vi "LVAPT_Git_Item_OnUpdateCommand.vi"(10 "Menu Item In":T1={"Menu Name"="", "Description"="", "Icon File Name"=path "", "Menu Tag"="", "Enabled"=TRUE, "Checked"=FALSE, "Separator"=FALSE, "Batchable"=TRUE, "Weight"=0, "Batch Mode (Ignored if Not Batchable)"=enum."Show If All Items Support Command", "Menu Location"=enum."<None>", "Exclude From Getting Started Window Menu"=FALSE}, 11 "Object":T2) -> (3 "Menu Item Out":T1={"Menu Name"="", "Description"="", "Icon File Name"=path "", "Menu Tag"="", "Enabled"=TRUE, "Checked"=FALSE, "Separator"=FALSE, "Batchable"=TRUE, "Weight"=0, "Batch Mode (Ignored if Not Batchable)"=enum."Show If All Items Support Command", "Menu Location"=enum."<None>", "Exclude From Getting Started Window Menu"=FALSE})   [LabVIEW 2019]
uses:
  <resource>/Framework/Providers/API/ItemRef.ctl
  <resource>/Framework/Providers/API/mxLvMenuItem.ctl
  <vilib>/Hampel Software Engineering/Git API/Git API/GIT-api.lvclass/GIT-api.ctl
  <vilib>/Hampel Software Engineering/Git API/Git API/Accessors/GIT-Set Working Dir.vi
  <vilib>/Utility/High Resolution Relative Seconds.vi
  <userlib>/_OpenG.lib/comparison/comparison.llb/Variant Changed__ogtk.vi
  <vilib>/Hampel Software Engineering/Git API/Git API/GIT-api.lvclass
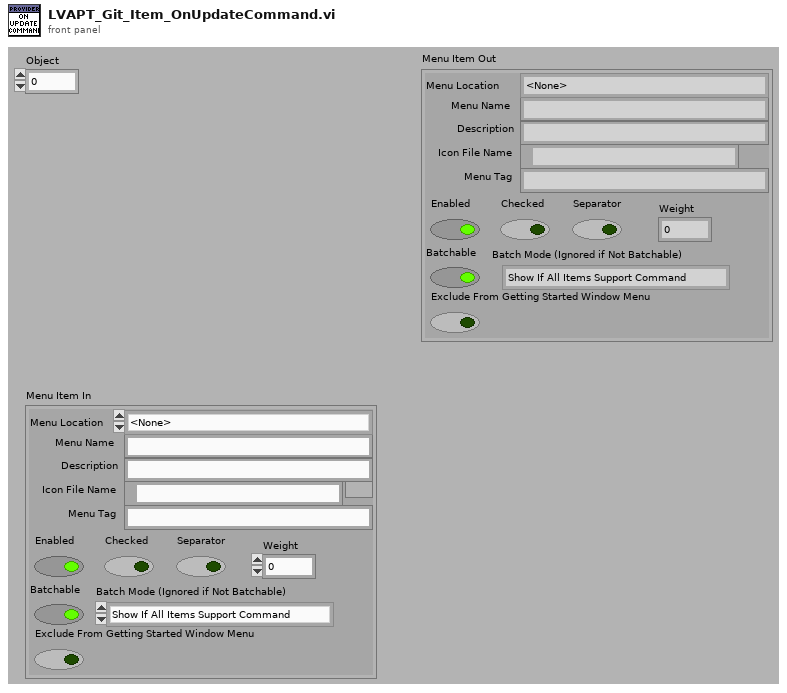
[diagram p1: front panel]
types:
  T1 = typedef "mxLvMenuItem.ctl" = cluster{"Menu Name":string, "Description":string, "Icon File Name":path, "Menu Tag":string, "Enabled":bool, "Checked":bool, "Separator":bool, "Batchable":bool, "Weight":i32, "Batch Mode (Ignored if Not Batchable)":enum32{"Show If All Items Support Command", "Show If Any Items Support Command"}, "Menu Location":enum32{"<None>", "Project", "Project / Build Specifications", "Tools", "Tools / Source Control", "Tools / Real-Time Module", "Help"}, "Exclude From Getting Started Window Menu":bool}
  T2 = typedef "ItemRef.ctl" = u64
  T3 = cluster{"current branch":string, "current commit":string, "Commit Info":string}
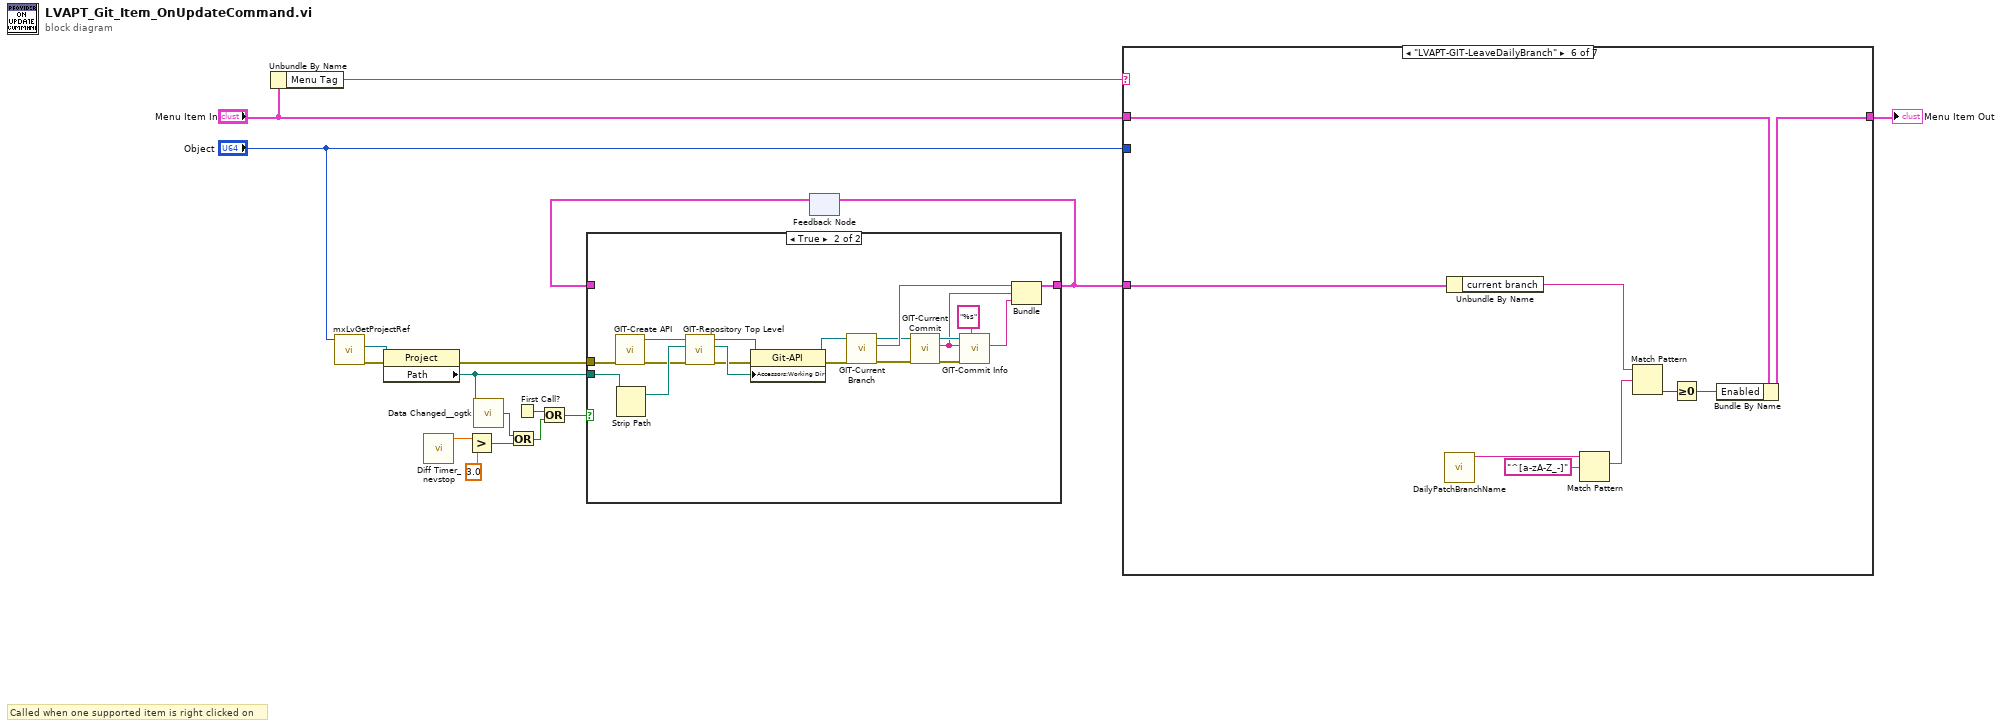
[diagram p0: block diagram]
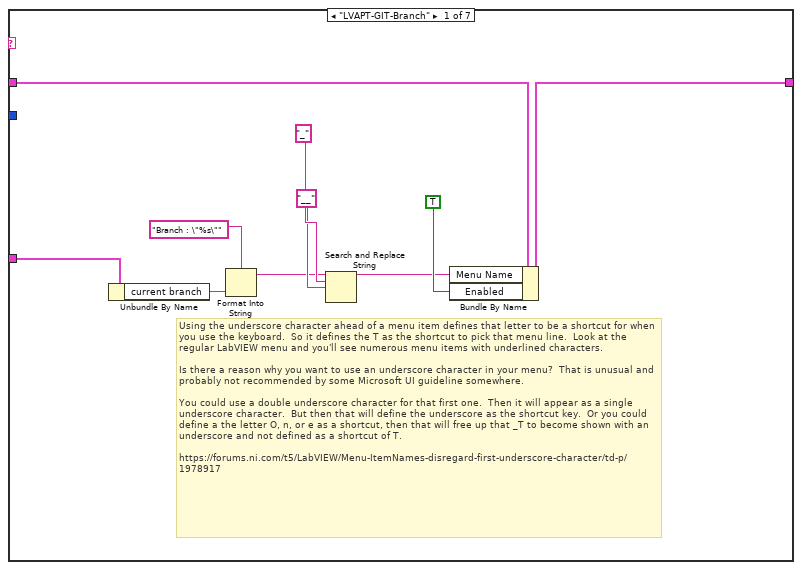
[diagram p3: hidden frame]
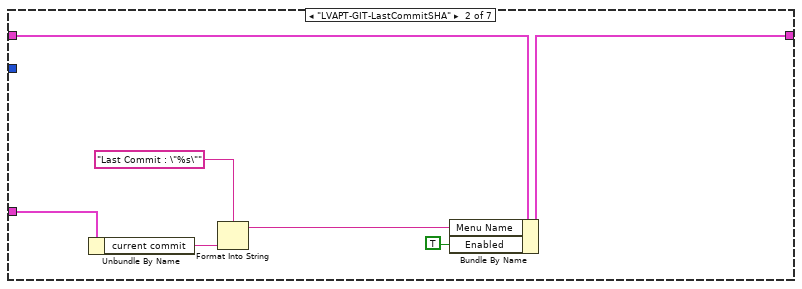
[diagram p4: hidden frame]
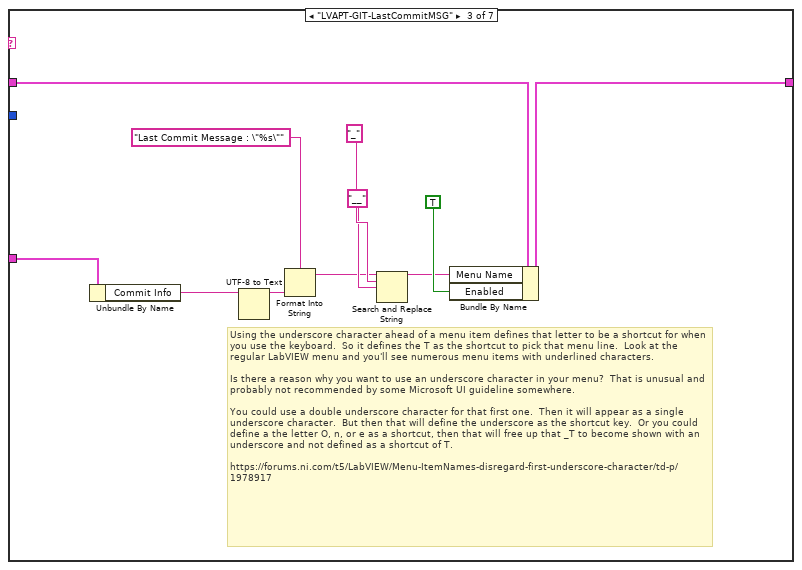
[diagram p5: hidden frame]
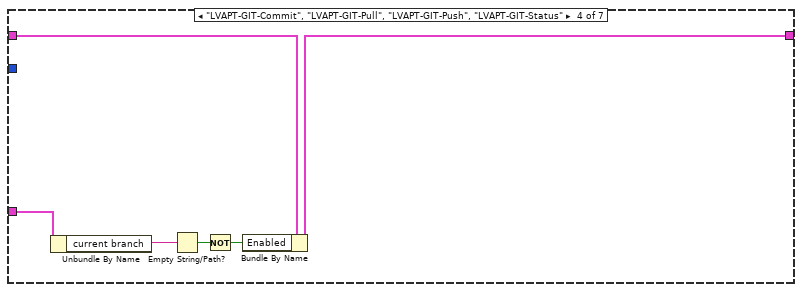
[diagram p6: hidden frame]
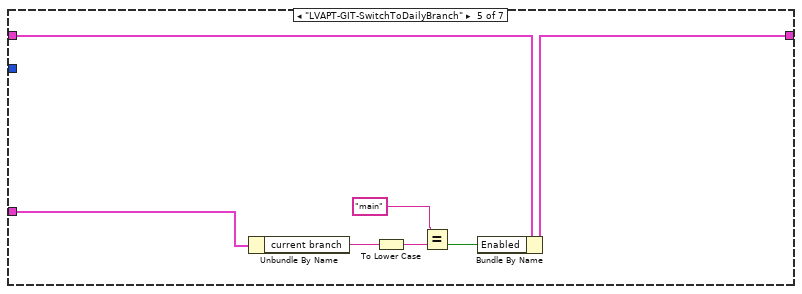
[diagram p7: hidden frame]
diagram:
  # "Called when one supported item is right clicked on"
  n1 = Unbundle By Name("Menu Item In") -> ("Menu Tag"=w17:string)
  n2 = call <resource>:"mxLvGetProjectRef.vi"("Item"="Object") -> ("error out"=w12:errorcluster, "Project Refnum"=w13:refnum<vi>)  [unwired: 8 in, 1 out]
  n3 = property class="Project"(reference=w13, error in=w12) -> (error out=w11:errorcluster, "Path"=w5:path)  [unwired: 1 out]
  n4 = call <userlib>:"Diff Timer_nevstop.vi"() -> ("time diff(s)"=w10:dbl)  [unwired: 10 in, 1 out]
  n5 = Greater?(x=w10, y=3.0) -> (0:w8:bool)
  n6 = call-poly <userlib>:"Data Changed__ogtk.vi"("Variant"=w5) -> ("Changed"=w4:bool)
  n7 = Or(x=w4, y=w8) -> (x .or. y?=w7:bool)
  n8 = First Call?() -> (First Call?: T/F=w6:bool)
  n9 = Or(x=w6, y=w7) -> (x .or. y?=w3:bool)
  n10 = feedback #1() -> (w2:T3)  [unwired: 1 in]
  n11 = case shown="True" w3 {
    tunnel: w11 -> [_ w29]
    tunnel: w5 -> [_ w28]
    tunnel: w2 -> [w18 _]
    tunnel: [w18 w26] -> w1
    frame False {
    }
    frame True {
      n12 = call <vilib>:"GIT-Create API.vi"("error in"=w29) -> ("error out"=w36:errorcluster, "git-api out"=w35:refnum<class "GIT-api.lvclass">)  [unwired: 9 in]
      n13 = Strip Path(path=w28) -> (stripped path=w37:path)  [unwired: 1 out]
      n14 = call <vilib>:"GIT-Repository Top Level.vi"("error in"=w36, "Current Path"=w37, "git-api in"=w35) -> ("error out"=w30:errorcluster, "Repo Top Level Path"=w32:path, "git-api out"=w31:refnum<class "GIT-api.lvclass">)  [unwired: 6 in]
      n15 = property class="Git-API"(reference=w31, error in=w30, "Accessors:Working Dir"=w32) -> (reference out=w33:refnum<class "GIT-api.lvclass">, error out=w34:errorcluster)
      n16 = call <vilib>:"GIT-Current Branch.vi"("error in"=w34, "git-api in"=w33) -> ("error out"=w24:errorcluster, "current branch"=w27:string, "git-api out"=w25:refnum<class "GIT-api.lvclass">)  [unwired: 7 in]
      n17 = call <vilib>:"GIT-Current Commit.vi"("error in"=w24, "git-api in"=w25) -> ("error out"=w21:errorcluster, "current commit"=w19:string, "git-api out"=w22:refnum<class "GIT-api.lvclass">)  [unwired: 7 in]
      n18 = call <vilib>:"GIT-Commit Info.vi"("Format String"="%s", "error in"=w21, "Commit"=w19, "git-api in"=w22) -> ("Commit Info"=w20:string)  [unwired: 5 in, 2 out]
      n19 = Bundle("current branch"=w27, "current commit"=w19, "Commit Info"=w20) -> (w26:T3)  [unwired: 1 in]
    }
  }
  n20 = feedback-in #1(w1) -> ()
  n21 = case shown="\"LVAPT-GIT-LeaveDailyBranch\"" w17 {
    tunnel: [w46 w53 w64 w70 w77 w86 w88] -> w16
    tunnel: "Menu Item In" -> [w47 w54 w65 w71 w78 w87 w88]
    tunnel: "Object" -> [_ _ _ _ _ _ _]
    tunnel: w1 -> [w38 w49 w56 w67 w73 w80 _]
    frame "LVAPT-GIT-Branch" {
      # "Using the underscore character ahead of a menu item defines that letter to be a shortcut for when you use the keyboard.  So it defines the T as the shortcut to pick that menu line.  Look at the regular LabVIEW menu and you'll see numerous menu items with underlined characters. \n\nIs there a reason why you want to use an underscore character in your menu?  That is unusual and probably not recommended by some Microsoft UI guideline somewhere.\n\nYou could use a double underscore character for that first one.  Then it will appear as a single underscore character.  But then that will define the underscore as the shortcut key.  Or you could define a the letter O, n, or e as a shortcut, then that will free up that _T to become shown with an underscore and not defined as a shortcut of T.\n\nhttps://forums.ni.com/t5/LabVIEW/Menu-ItemNames-disregard-first-underscore-character/td-p/1978917"
      n22 = Unbundle By Name(w38) -> ("current branch"=w39:string)
      n23 = Format Into String(format string="Branch : \"%s\"" ("string"), w39) -> (resulting string=w40:string)  [unwired: 2 in, 1 out]
      n24 = Search and Replace String(input string=w40, search string="_", replace string="__" ("replace string (\"\")")) -> (result string=w43:string)  [unwired: 5 in, 3 out]
      n25 = Bundle By Name(cluster=w47, "Menu Name"=w43, "Enabled"=TRUE) -> (w46:T1)
    }
    frame "LVAPT-GIT-LastCommitSHA" {
      n26 = Unbundle By Name(w49) -> ("current commit"=w48:string)
      n27 = Format Into String(format string="Last Commit : \"%s\"" ("string"), w48) -> (resulting string=w50:string)  [unwired: 2 in, 1 out]
      n28 = Bundle By Name(cluster=w54, "Menu Name"=w50, "Enabled"=TRUE) -> (w53:T1)
    }
    frame "LVAPT-GIT-LastCommitMSG" {
      # "Using the underscore character ahead of a menu item defines that letter to be a shortcut for when you use the keyboard.  So it defines the T as the shortcut to pick that menu line.  Look at the regular LabVIEW menu and you'll see numerous menu items with underlined characters. \n\nIs there a reason why you want to use an underscore character in your menu?  That is unusual and probably not recommended by some Microsoft UI guideline somewhere.\n\nYou could use a double underscore character for that first one.  Then it will appear as a single underscore character.  But then that will define the underscore as the shortcut key.  Or you could define a the letter O, n, or e as a shortcut, then that will free up that _T to become shown with an underscore and not defined as a shortcut of T.\n\nhttps://forums.ni.com/t5/LabVIEW/Menu-ItemNames-disregard-first-underscore-character/td-p/1978917"
      n29 = Unbundle By Name(w56) -> ("Commit Info"=w55:string)
      n30 = UTF-8 to Text(11:w55) -> (3:w57:string)  [unwired: 2 in, 1 out]
      n31 = Format Into String(format string="Last Commit Message : \"%s\"" ("string"), w57) -> (resulting string=w58:string)  [unwired: 2 in, 1 out]
      n32 = Search and Replace String(input string=w58, search string="_", replace string="__" ("replace string (\"\")")) -> (result string=w61:string)  [unwired: 5 in, 3 out]
      n33 = Bundle By Name(cluster=w65, "Menu Name"=w61, "Enabled"=TRUE) -> (w64:T1)
    }
    frame "LVAPT-GIT-Commit", "LVAPT-GIT-Pull", "LVAPT-GIT-Push", "LVAPT-GIT-Status" {
      n34 = Unbundle By Name(w67) -> ("current branch"=w66:string)
      n35 = Empty String/Path?(string/path=w66) -> (empty?=w69:bool)
      n36 = Not(x=w69) -> (.not. x?=w68:bool)
      n37 = Bundle By Name(cluster=w71, "Enabled"=w68) -> (w70:T1)
    }
    frame "LVAPT-GIT-SwitchToDailyBranch" {
      n38 = Unbundle By Name(w73) -> ("current branch"=w72:string)
      n39 = To Lower Case(string=w72) -> (all lower case string=w74:string)
      n40 = Equal?(x="main", y=w74) -> (x = y?=w76:bool)
      n41 = Bundle By Name(cluster=w78, "Enabled"=w76) -> (w77:T1)
    }
    frame "LVAPT-GIT-LeaveDailyBranch" {
      n42 = call "DailyPatchBranchName.vi"() -> ("DailyPatchBranchName"=w83:string)  [unwired: 11 in]
      n43 = Unbundle By Name(w80) -> ("current branch"=w79:string)
      n44 = Match Pattern(string=w83, regular expression="^[a-zA-Z_-]") -> (match substring=w81:string)  [unwired: 1 in, 3 out]
      n45 = Match Pattern(string=w79, regular expression=w81) -> (offset past match=w85:i32)  [unwired: 1 in, 3 out]
      n46 = Greater Or Equal To 0?(x=w85) -> (x >= 0?=w84:bool)
      n47 = Bundle By Name(cluster=w87, "Enabled"=w84) -> (w86:T1)
    }
    frame Default {
    }
  }
  "Menu Item Out" <- w16
